vi "10_1.vi"() -> ()   [LabVIEW 2021, in "2022.lvlib"]
uses:
  2022.lvlib
panel:
  out "Array 3":string[][](array[string])
  out "Array 2":i32[](array[numeric])
  out "sum":i32
  out "Array":i32[](array[numeric])
  out "output 2":i32
  out "Numeric":i32
  out "delimiter":string
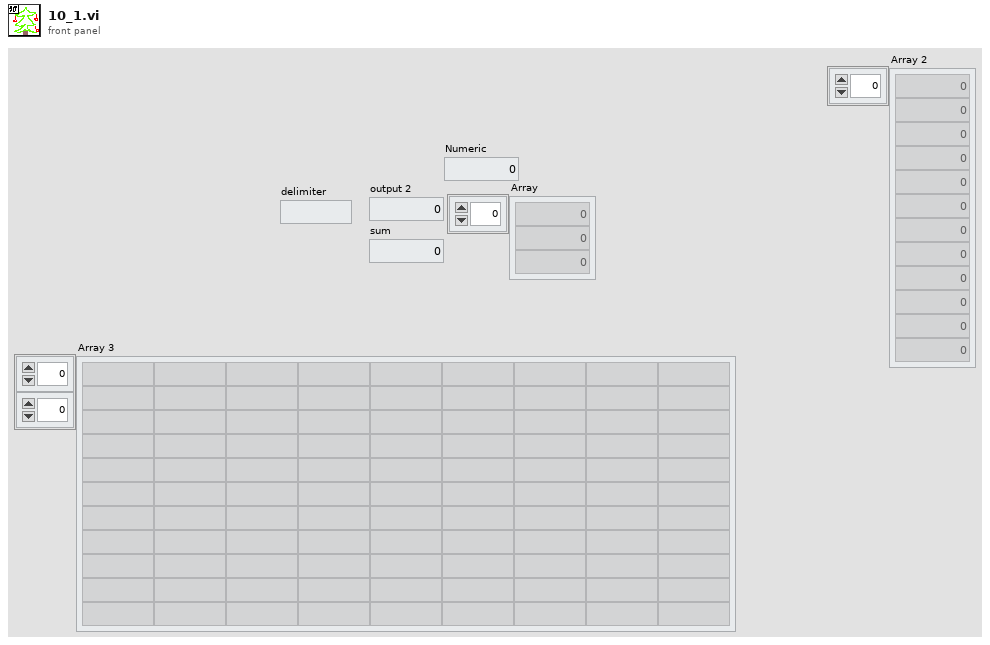
[diagram p1: front panel]
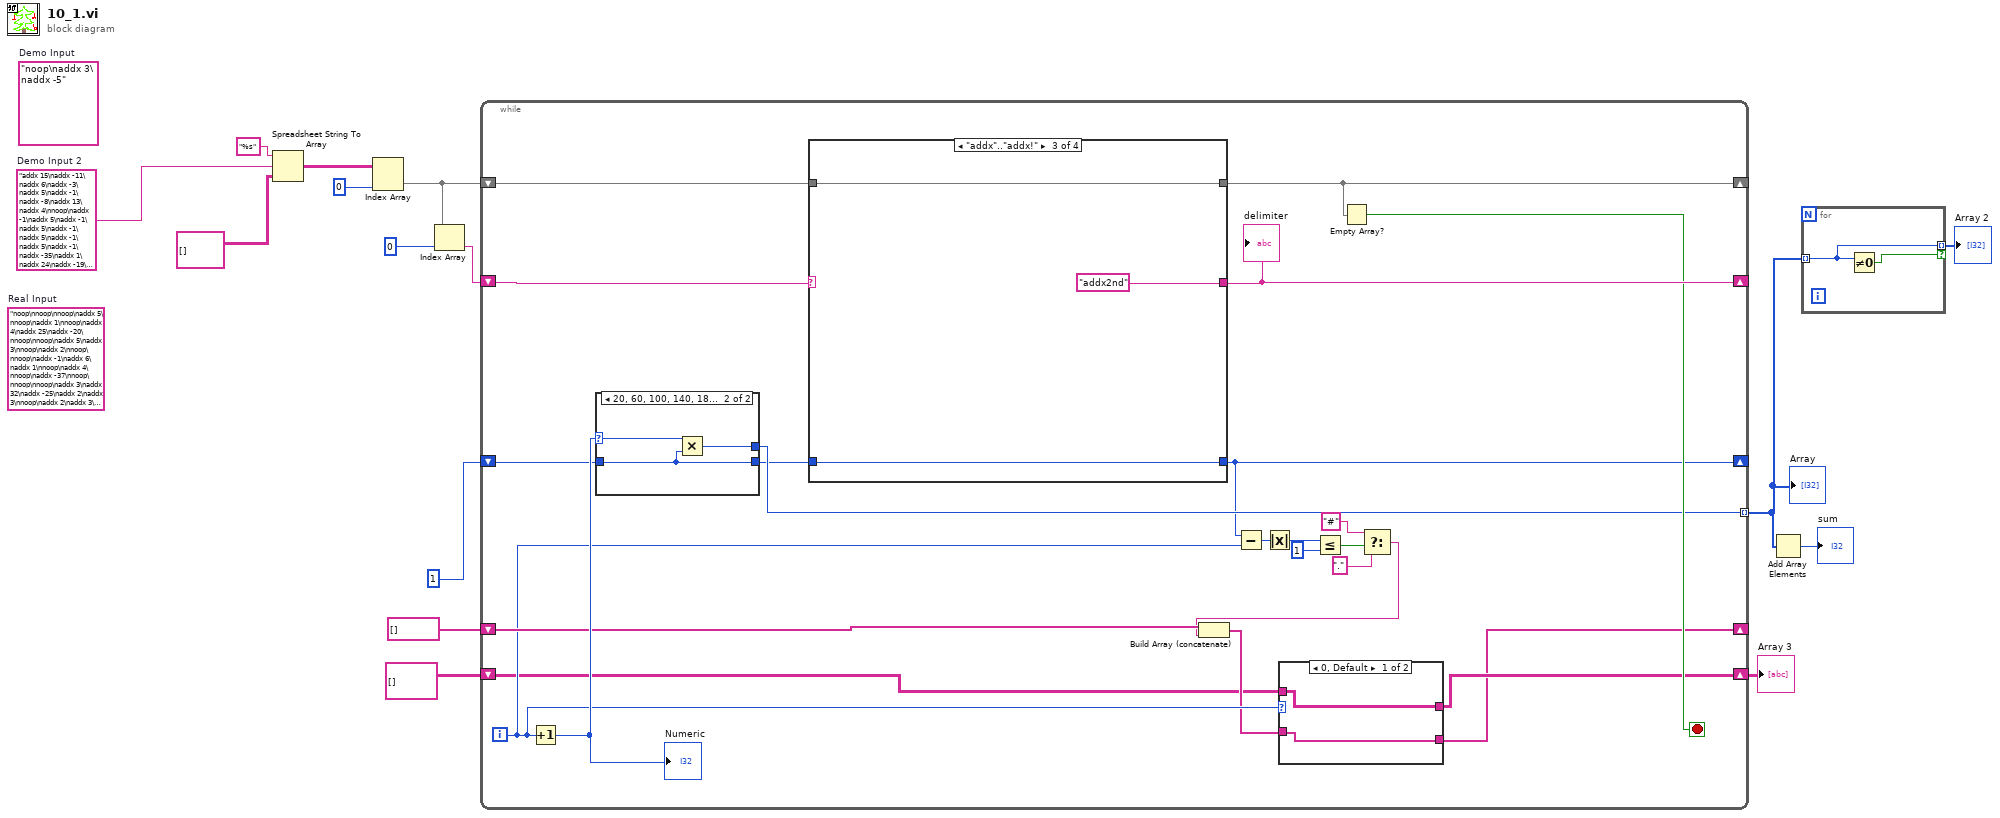
[diagram p0: block diagram]
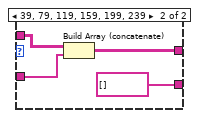
[diagram p2: hidden frame]
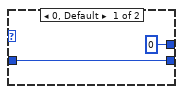
[diagram p3: hidden frame]
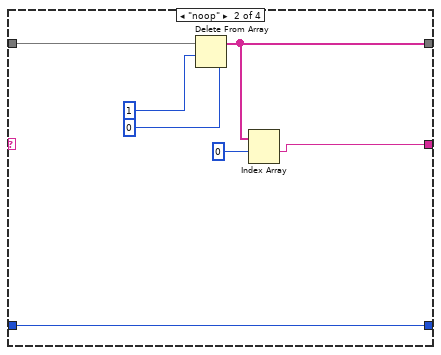
[diagram p5: hidden frame]
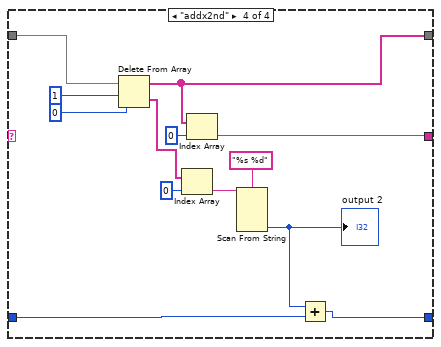
[diagram p6: hidden frame]
diagram:
  w4 = "addx 15\naddx -11\naddx 6\naddx -3\naddx 5\naddx -1\naddx -8\naddx 13\naddx 4\nnoop\naddx -1\naddx 5\naddx -1\naddx 5\naddx -1\naddx 5\naddx -1\naddx 5\naddx -1\naddx -35\naddx 1\naddx 24\naddx -19\naddx 1\naddx 16\naddx -11\nnoop\nnoop\naddx 21\naddx -15\nnoop\nnoop\naddx -3\naddx 9\naddx 1\naddx -3\naddx 8\naddx 1\naddx 5\nnoop\nnoop\nnoop\nnoop\nnoop\naddx -36\nnoop\naddx 1\naddx 7\nnoop\nnoop\nnoop\naddx 2\naddx 6\nnoop\nnoop\nnoop\nnoop\nnoop\naddx 1\nnoop\nnoop\naddx 7\naddx 1\nnoop\naddx -13\naddx 13\naddx 7\nnoop\naddx 1\naddx -33\nnoop\nnoop\nnoop\naddx 2\nnoop\nnoop\nnoop\naddx 8\nnoop\naddx -1\naddx 2\naddx 1\nnoop\naddx 17\naddx -9\naddx 1\naddx 1\naddx -3\naddx 11\nnoop\nnoop\naddx 1\nnoop\naddx 1\nnoop\nnoop\naddx -13\naddx -19\naddx 1\naddx 3\naddx 26\naddx -30\naddx 12\naddx -1\naddx 3\naddx 1\nnoop\nnoop\nnoop\naddx -9\naddx 18\naddx 1\naddx 2\nnoop\nnoop\naddx 9\nnoop\nnoop\nnoop\naddx -1\naddx 2\naddx -37\naddx 1\naddx 3\nnoop\naddx 15\naddx -21\naddx 22\naddx -6\naddx 1\nnoop\naddx 2\naddx 1\nnoop\naddx -10\nnoop\nnoop\naddx 20\naddx 1\naddx 2\naddx 2\naddx -6\naddx -11\nnoop\nnoop\nnoop"  # Demo Input 2
  (unwired) "noop\nnoop\nnoop\naddx 5\nnoop\naddx 1\nnoop\naddx 4\naddx 25\naddx -20\nnoop\nnoop\naddx 5\naddx 3\nnoop\naddx 2\nnoop\nnoop\naddx -1\naddx 6\naddx 1\nnoop\naddx 4\nnoop\naddx -37\nnoop\nnoop\nnoop\naddx 3\naddx 32\naddx -25\naddx 2\naddx 3\nnoop\naddx 2\naddx 3\nnoop\naddx 2\naddx 2\naddx -24\naddx 25\naddx 5\naddx 2\naddx 8\naddx -23\naddx 18\naddx 5\naddx -39\naddx 11\naddx -9\naddx 6\naddx -2\naddx 5\naddx 4\naddx -4\naddx 3\naddx 5\naddx 2\nnoop\naddx -1\naddx 6\naddx -21\naddx 22\naddx 3\naddx 1\naddx 5\nnoop\nnoop\naddx -35\nnoop\nnoop\nnoop\nnoop\naddx 37\naddx -33\nnoop\naddx 6\naddx 2\naddx -1\naddx 3\naddx 1\naddx 5\naddx 2\naddx -19\naddx 21\naddx 1\naddx 5\naddx -31\naddx 36\nnoop\naddx 3\naddx -2\naddx -38\nnoop\nnoop\naddx 7\naddx 14\naddx -4\naddx -7\naddx 5\naddx 2\naddx 12\naddx -15\naddx 6\naddx 2\naddx 5\naddx -27\naddx 25\naddx 5\nnoop\naddx 7\naddx -2\naddx 5\naddx -40\nnoop\naddx 7\nnoop\naddx -1\naddx 2\naddx 5\naddx -1\naddx 1\naddx 2\naddx 7\nnoop\naddx -2\nnoop\naddx 3\naddx 2\naddx 7\nnoop\nnoop\naddx 1\nnoop\nnoop\naddx 3\naddx 1\nnoop\nnoop\nnoop"  # Real Input
  (unwired) "noop\naddx 3\naddx -5"  # Demo Input
  n1 = Spreadsheet String To Array(format string="%s", spreadsheet string=w4, array type (2D Dbl)=string[][] []) -> (array=w13:string[][])  [unwired: 1 in]
  n2 = Index Array(array=w13, index (col)=0 ("index (row)")) -> (element=w12:string[])  [unwired: 1 in]
  n3 = Index Array(array=w12, index=0) -> (element=w11:string)
  n4 = while {
    shift-right: [w35] -> _
    shift-left: w12 -> [w38]
    shift-right: [w36] -> _
    shift-left: w11 -> [w37]
    shift-right: [w29] -> _
    shift-left: 1 ("Numeric") -> [w31]
    tunnel: [w32] -> w6 mode=indexing
    shift-right: [w16] -> _
    shift-left: string[] [] -> [w25]
    shift-right: [w17] -> w1
    shift-left: string[][] [] -> [w18]
    i -> [w20]
    stop <- w34 stop-if-true
    n5 = Increment(x=w20) -> (x+1=w33:i32)
    "Numeric" <- w33
    n6 = case shown="20, 60, 100, 140, 180, 220" w33 {
      selector: w33 -> [_ w49]
      tunnel: [w46 w47] -> w30
      tunnel: w31 -> [w46 w47]
      tunnel: [0 w48] -> w32
      frame 0, Default {
      }
      frame 20, 60, 100, 140, 180, 220 {
        n7 = Multiply(x=w49, y=w47) -> (x*y=w48:i32)
      }
    }
    n8 = case shown="\"addx\"..\"addx!\"" w37 {
      selector: w37 -> [w51 _ _ _]
      tunnel: w38 -> [w52 w59 w62 w72]
      tunnel: [w52 w55 w62 w71] -> w35
      tunnel: [w51 w54 "addx2nd" ("delimiter") w69] -> w36
      tunnel: w30 -> [w50 w53 w60 w67]
      tunnel: [w50 w53 w60 w66] -> w29
      frame "False", Default {
      }
      frame "noop" {
        n9 = Delete From Array(array=w59, length=1, index=0) -> (array with subset deleted=w55:string[])  [unwired: 1 out]
        n10 = Index Array(array=w55, index #1=0 ("index")) -> (element #1=w54:string)  [unwired: 1 in, 1 out]
      }
      frame "addx".."addx!" {
      }
      frame "addx2nd" {
        n11 = Delete From Array(array=w72, length=1, index=0) -> (deleted portion=w64:string[], array with subset deleted=w71:string[])
        n12 = Index Array(array=w64, index=0) -> (element=w63:string)
        n13 = Index Array(array=w71, index=0) -> (element=w69:string)
        n14 = Scan From String(format string="%s %d", input string=w63) -> (output 2=w68:i32)  [unwired: 5 in, 3 out]
        "output 2" <- w68
        n15 = Add(x=w68, y=w67) -> (x+y=w66:i32)
      }
    }
    "delimiter" <- w36
    n16 = Subtract(x=w29, y=w20) -> (x-y=w27:i32)
    n17 = Absolute Value(x=w27) -> (abs(x)=w28:i32)
    n18 = Less Or Equal?(x=w28, y=1) -> (x <= y?=w24:bool)
    n19 = Empty Array?(array=w35) -> (empty?=w34:bool)
    n20 = Select(t="#" ("delimiter"), s=w24, f=".") -> (s? t:f=w21:string)
    n21 = Build Array (concatenate)(w25, w21) -> (w19:string[])
    n22 = case shown="0, Default" w20 {
      tunnel: w19 -> [w39 w43]
      tunnel: w18 -> [w40 w44]
      tunnel: [w40 w42] -> w17
      tunnel: [w39 string[] []] -> w16
      frame 0, Default {
      }
      frame 39, 79, 119, 159, 199, 239 {
        n23 = Build Array (concatenate)(w44, w43) -> (w42:string[][])
      }
    }
  }
  "Array" <- w6
  "Array 3" <- w1
  n24 = Add Array Elements(numeric array=w6) -> (sum=→"sum":i32)
  n25 = for {
    tunnel: w6 -> [w77] mode=indexing
    tunnel: [w77] -> w5 mode=indexing if=w76
    n26 = Not Equal To 0?(x=w77) -> (x != 0?=w76:bool)
  }
  "Array 2" <- w5
